vi "listen.vi"(6 "timeout ms (10000)":i32=10000, 8 "error in":errorcluster, 11 "TCP server in":refnum<class "TCP server.lvclass">) -> (0 "error out":errorcluster, 1 "valid?":bool, 2 "new connection":refnum<class "connection maintainer.lvclass">, 3 "TCP server out":refnum<class "TCP server.lvclass">, 5 "client ID":string)   [LabVIEW 2015, in "TCP server.lvclass"]
uses:
  TCP server.lvclass
  connection/connection maintainer.lvclass
  TCP server.lvclass/TCP server.ctl
  TCP connection/TCP connection.lvclass/TCP connection.ctl
  TCP connection/TCP connection.lvclass
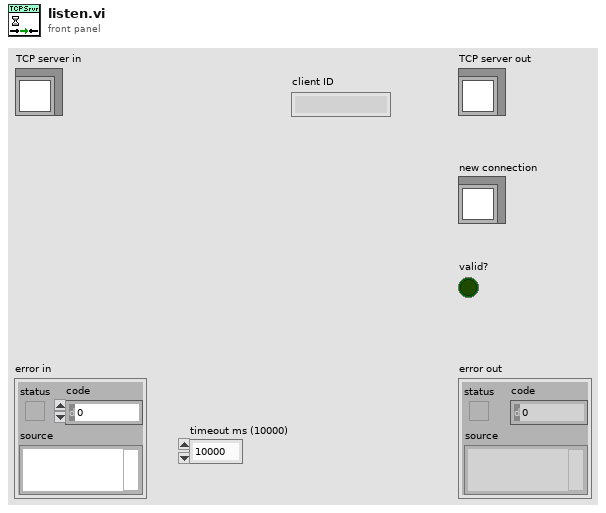
[diagram p1: front panel]
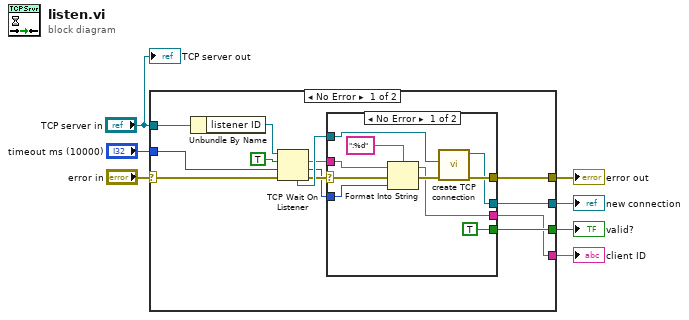
[diagram p0: block diagram]
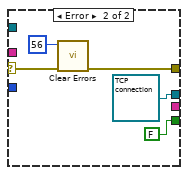
[diagram p2: hidden frame]
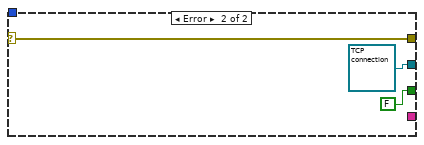
[diagram p3: hidden frame]
diagram:
  n1 = case shown="No Error" "error in" {
    selector: "error in" -> [w14 w38]
    tunnel: "timeout ms (10000)" -> [w19 _]
    tunnel: "TCP server in" -> [w15 _]
    tunnel: [w13 w38] -> w4
    tunnel: [w11 FALSE] -> w3
    tunnel: [w12 refnum<class "TCP connection.lvclass"> refnum ("TCP connection out")] -> w2
    tunnel: [w10 _] -> w1
    frame No Error {
      n2 = Unbundle By Name(w15) -> ("listener ID"=w16:refnum<k5>)
      n3 = TCP Wait On Listener(8:w14, 9:w19, 10:TRUE ("resolve remote address (T)"), 11:w16) -> (0:w17:errorcluster, 1:w8:u16, 2:w9:string, 4:w18:refnum<k5>)  [unwired: 1 out]
      n4 = case shown="No Error" w17 {
        selector: w17 -> [w29 w33]
        tunnel: w18 -> [w30 _]
        tunnel: [w28 w32] -> w13
        tunnel: [w27 refnum<class "TCP connection.lvclass"> refnum ("TCP connection out")] -> w12
        tunnel: [TRUE FALSE] -> w11
        tunnel: [w24 _] -> w10
        tunnel: w9 -> [w23 _]
        tunnel: w8 -> [w22 _]
        frame No Error {
          n5 = Format Into String(format string=":%d", initial string=w23, error in=w29, w22) -> (resulting string=w24:string, error out=w25:errorcluster)
          n6 = call "create TCP connection.vi"("error in"=w25, "connection"=w30) -> ("error out"=w28:errorcluster, "TCP connection out"=w27:refnum<class "TCP connection.lvclass">)  [unwired: 8 in]
        }
        frame Error {
          n7 = call <vilib>:"Clear Errors.vi"("error in (no error)"=w33, "specific error code to clear (0: all)"=56) -> ("error out"=w32:errorcluster)  [unwired: 4 in, 1 out]
        }
      }
    }
    frame Error {
    }
  }
  "error out" <- w4
  "new connection" <- w2
  "valid?" <- w3
  "client ID" <- w1
  "TCP server out" <- "TCP server in"
